vi "FPGA_OP.vi"(5 "Origin_Value":u32, 6 "OP_Offset":u32, 7 "Offset":u32, 8 "Error_In":errorcluster, 11 "VISA_Rsrc_In":refnum<visa-resource-name>) -> (0 "Error_Out":errorcluster, 3 "VISA_Rsrc_Out":refnum<visa-resource-name>)   [LabVIEW 2018]
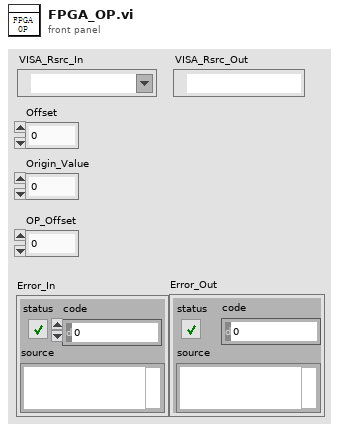
[diagram p1: front panel]
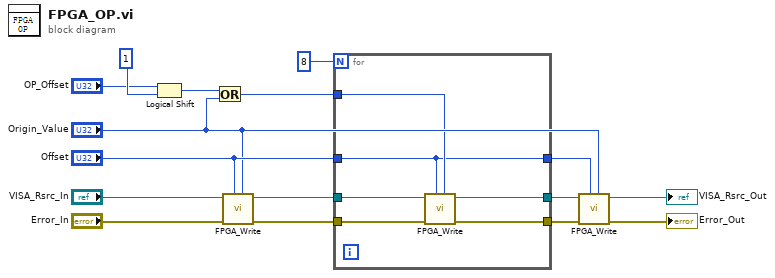
[diagram p0: block diagram]
diagram:
  n1 = Logical Shift(y="OP_Offset", x=u32 1) -> (x << y=w14:u32)
  n2 = Or(x=w14, y="Origin_Value") -> (x .or. y?=w13:u32)
  n3 = call "FPGA_Write.vi"("Value"="Origin_Value", "Offset"="Offset", "Error_In"="Error_In", "VISA_Rsrc_In"="VISA_Rsrc_In") -> ("Error_Out"=w7:errorcluster, "VISA_Rsrc_Out"=w8:refnum<visa-resource-name>)  [unwired: 6 in]
  n4 = for {
    N: 8 -> [_]
    tunnel: w8 -> [w22]
    tunnel: "Offset" -> [w17]
    tunnel: w13 -> [w21]
    tunnel: w7 -> [w20]
    tunnel: [w19] -> w6
    tunnel: [w18] -> w5
    tunnel: [w17] -> w4
    n5 = call "FPGA_Write.vi"("Value"=w21, "Offset"=w17, "Error_In"=w20, "VISA_Rsrc_In"=w22) -> ("Error_Out"=w18:errorcluster, "VISA_Rsrc_Out"=w19:refnum<visa-resource-name>)  [unwired: 6 in]
  }
  n6 = call "FPGA_Write.vi"("Value"="Origin_Value", "Offset"=w4, "Error_In"=w5, "VISA_Rsrc_In"=w6) -> ("Error_Out"=→"Error_Out":errorcluster, "VISA_Rsrc_Out"=→"VISA_Rsrc_Out":refnum<visa-resource-name>)  [unwired: 6 in]
